vi "Interp2D.vi"(6 "method":i32(ring)=3 items=["nearest", "bilinear", "bicubic", "bicubic spline"], 7 "Fixed Axis":T1, 9 "Interpolation Points":i32=100, 10 "Meas maxima":dbl[](array[numeric]) format="%.1f", 11 "Measured Points":dbl[][](array[numeric]) format="%.2f") -> (1 "Yi":dbl, 2 "Xi":dbl, 3 "max value":dbl)   [LabVIEW 2011]
uses:
  <vilib>/Math Plots/3D Math Plots/3D Surface/3D Surface XCtrl/3D Surface.xctl
  Gen Trav/Route mapping/Axis.ctl
  <vilib>/Analysis/1siggen.llb/Ramp Pattern by Samples.vi
  <vilib>/gmath/interp.llb/Create Mesh Grid (2D) (x,y arrays).vi
  <vilib>/gmath/interp.llb/Interpolate 2D (2d X,Y).vi
  <vilib>/Math Plots/3D Math Plots/3D Surface/3D Surface Datatype/Public/Plot Helper (Matrix).vi
  <vilib>/gmath/NI_Gmath.lvlib
  <vilib>/Analysis/NI_AALBase.lvlib
  <vilib>/Math Plots/3D Math Plots/3D Surface/3D Surface Datatype/3D Surface Datatype.lvclass
panel:
  out "Interpolated Surface":refnum<class "3D Plot Datatype.lvclass">[](xcontrol)
  out "Input Surface":refnum<class "3D Plot Datatype.lvclass">[](xcontrol)
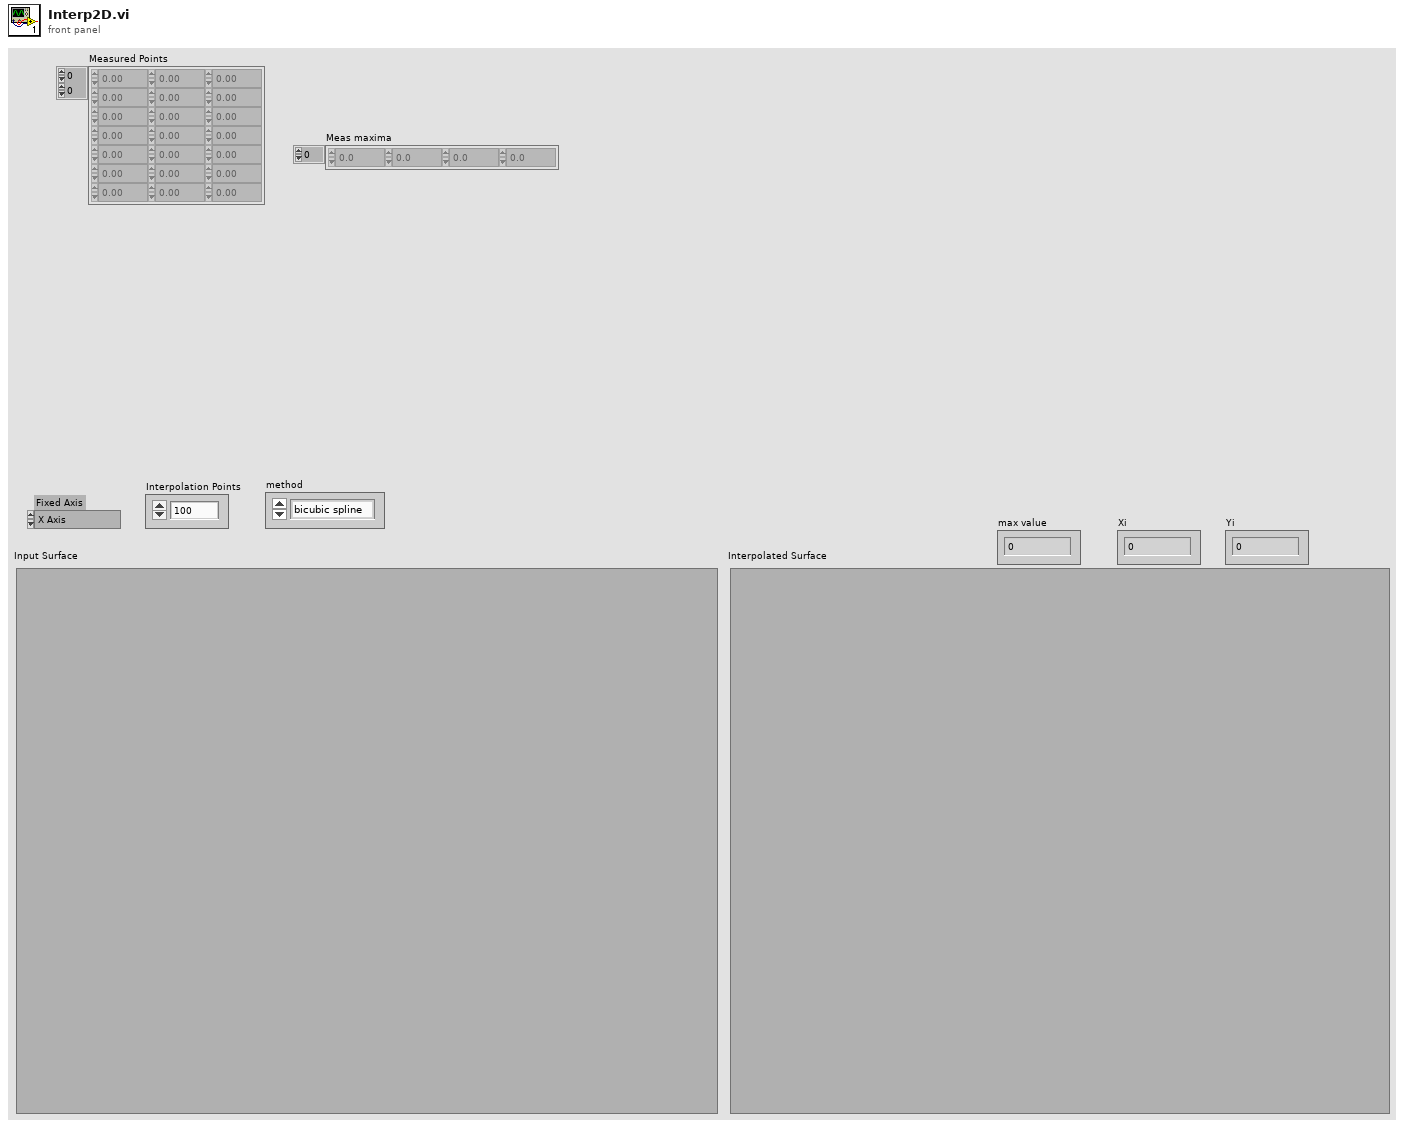
[diagram p1: front panel]
types:
  T1 = typedef "Axis.ctl" = enum16{"X Axis", "X Axis -ve", "Y Axis", "Y Axis -ve", "Z Axis", "Z Axis -ve"}
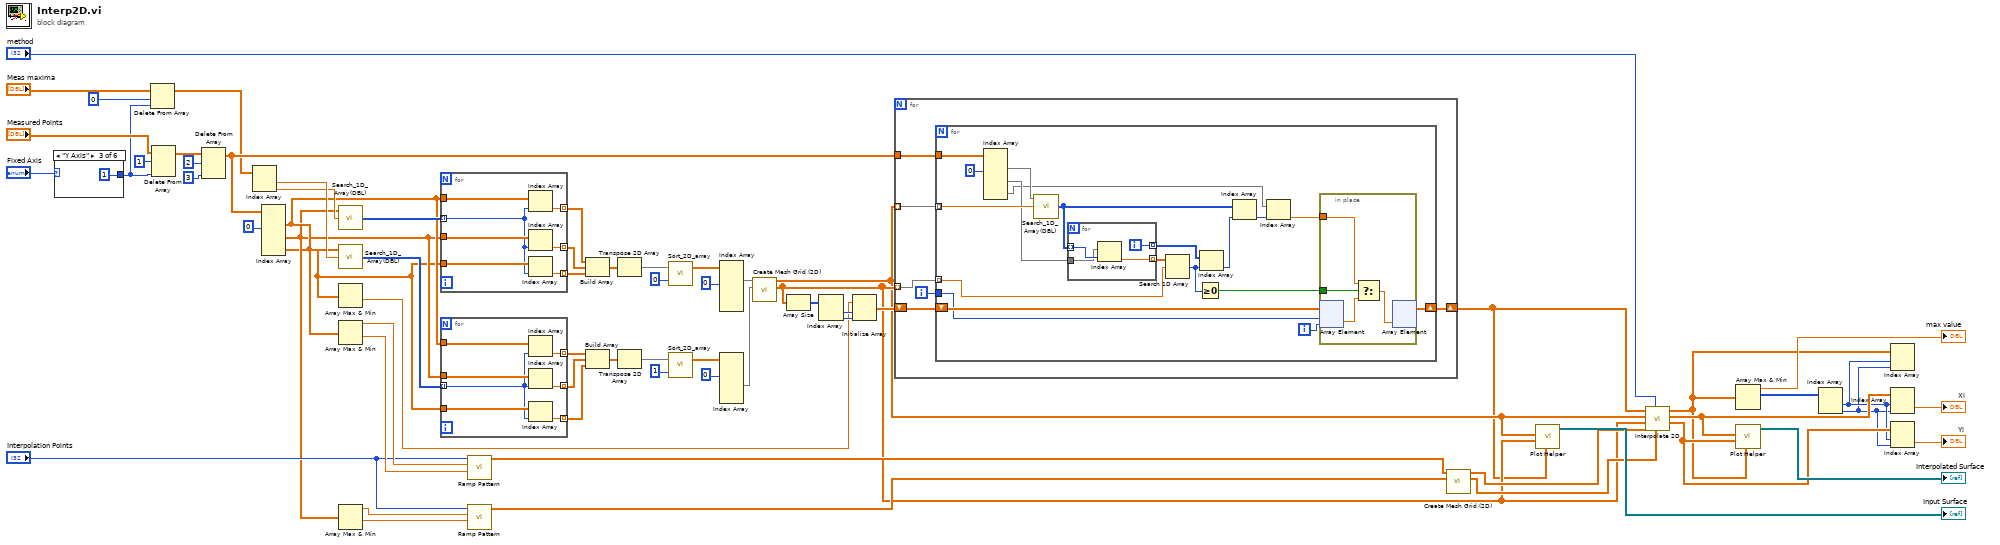
[diagram p0: block diagram]
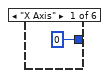
[diagram p2: hidden frame]
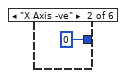
[diagram p3: hidden frame]
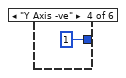
[diagram p4: hidden frame]
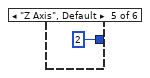
[diagram p5: hidden frame]
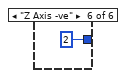
[diagram p6: hidden frame]
diagram:
  n1 = case shown="\"Y Axis\"" "Fixed Axis" {
    tunnel: [0 ("index") 0 ("index") 1 ("index") 1 ("index") 2 ("index") 2 ("index")] -> w1
    frame "X Axis" {
    }
    frame "X Axis -ve" {
    }
    frame "Y Axis" {
    }
    frame "Y Axis -ve" {
    }
    frame "Z Axis", Default {
    }
    frame "Z Axis -ve" {
    }
  }
  n2 = Delete From Array(array="Meas maxima", length=0, index=w1) -> (array with subset deleted=w3:dbl[])  [unwired: 1 out]
  n3 = Delete From Array(array="Measured Points", length=1, index (col)=w1) -> (array with subset deleted=w65:dbl[][])  [unwired: 1 in, 1 out]
  n4 = Delete From Array(array=w65, length=2, index (col)=3 ("disabled index (col)")) -> (array with subset deleted=w16:dbl[][])  [unwired: 1 in, 1 out]
  n5 = Index Array(array=w3) -> (element #1=w55:dbl, element #2=w53:dbl)  [unwired: 2 in]
  n6 = Index Array(array=w16, index (col) #1=0 ("disabled index (col)")) -> (element #1=w41:dbl[], element #2=w40:dbl[], element #3=w15:dbl[])  [unwired: 5 in]
  n7 = call "Search_1D_Array(DBL).vi"("Array"=w40, "Element Data"=w53) -> ("Indicies of Elements"=w52:i32[])  [unwired: 6 in, 1 out]
  n8 = call "Search_1D_Array(DBL).vi"("Array"=w41, "Element Data"=w55) -> ("Indicies of Elements"=w57:i32[])  [unwired: 6 in, 1 out]
  n9 = Array Max & Min(array=w15) -> (min value=w14:dbl)  [unwired: 3 out]
  n10 = Array Max & Min(array=w41) -> (max value=w46:dbl, min value=w45:dbl)  [unwired: 2 out]
  n11 = Array Max & Min(array=w40) -> (max value=w42:dbl, min value=w44:dbl)  [unwired: 2 out]
  n12 = for {
    tunnel: w52 -> [w73] mode=indexing
    tunnel: w41 -> [w79]
    tunnel: w15 -> [w78]
    tunnel: [w77] -> w31 mode=indexing
    tunnel: [w76] -> w50 mode=indexing
    tunnel: [w75] -> w49 mode=indexing
    tunnel: w40 -> [w74]
    n13 = Index Array(array=w79, index=w73) -> (element=w77:dbl)
    n14 = Index Array(array=w74, index=w73) -> (element=w75:dbl)
    n15 = Index Array(array=w78, index=w73) -> (element=w76:dbl)
  }
  n16 = for {
    tunnel: w57 -> [w80] mode=indexing
    tunnel: w41 -> [w86]
    tunnel: w15 -> [w85]
    tunnel: [w84] -> w39 mode=indexing
    tunnel: [w83] -> w54 mode=indexing
    tunnel: [w82] -> w38 mode=indexing
    tunnel: w40 -> [w81]
    n17 = Index Array(array=w86, index=w80) -> (element=w84:dbl)
    n18 = Index Array(array=w81, index=w80) -> (element=w82:dbl)
    n19 = Index Array(array=w85, index=w80) -> (element=w83:dbl)
  }
  n20 = call-poly <vilib>:"Ramp Pattern.vi"("start"=w45, "end"=w46, "samples"="Interpolation Points") -> ("Ramp Pattern"=w25:dbl[])  [unwired: 7 in, 1 out]
  n21 = call-poly <vilib>:"Ramp Pattern.vi"("start"=w44, "end"=w42, "samples"="Interpolation Points") -> ("Ramp Pattern"=w24:dbl[])  [unwired: 7 in, 1 out]
  n22 = Build Array(w31, w49, w50) -> (w51:dbl[][])
  n23 = Build Array(w39, w38, w54) -> (w56:dbl[][])
  n24 = Transpose 2D Array(2D array=w51) -> (transposed array=w47:dbl[][])
  n25 = Transpose 2D Array(2D array=w56) -> (transposed array=w60:dbl[][])
  n26 = call "Sort_2D_array.vi"("Column index to sort on"=0, "unsorted array"=w47) -> ("sorted array"=w32:dbl[][])  [unwired: 1 out]
  n27 = call "Sort_2D_array.vi"("Column index to sort on"=1, "unsorted array"=w60) -> ("sorted array"=w33:dbl[][])  [unwired: 1 out]
  n28 = Index Array(array=w32, index (col) #1=0 ("disabled index (col)")) -> (element #1=w30:dbl[])  [unwired: 5 in, 2 out]
  n29 = Index Array(array=w33, index (col) #1=0 ("disabled index (col)")) -> (element #2=w29:dbl[])  [unwired: 5 in, 2 out]
  n30 = call-poly <vilib>:"Create Mesh Grid (2D).vi"("y domain"=w29, "x domain"=w30) -> ("Y"=w21:dbl[][], "X"=w20:dbl[][])  [unwired: 7 in, 1 out]
  n31 = Array Size(array=w21) -> (size(s)=w37:i32[])
  n32 = Index Array(array=w37) -> (element #1=w36:i32, element #2=w35:i32)  [unwired: 2 in]
  n33 = Initialize Array(w14, w36, w35) -> (w34:dbl[][])
  n34 = for {
    tunnel: w20 -> [w92] mode=indexing
    tunnel: w21 -> [w91] mode=indexing
    tunnel: w16 -> [w90]
    shift-right: [w87] -> w17
    shift-left: w34 -> [w89]
    i -> [w88]
    n35 = for {
      tunnel: w92 -> [w109] mode=indexing
      tunnel: w91 -> [w107] mode=indexing
      tunnel: w90 -> [w111]
      shift-right: [w105] -> w87
      shift-left: w89 -> [w106]
      tunnel: w88 -> [w99]
      i -> [w98]
      n36 = Index Array(array=w111, index (col) #1=0 ("disabled index (col)")) -> (element #1=w108:dbl[], element #2=w104:dbl[], element #3=w102:dbl[])  [unwired: 5 in]
      n37 = call "Search_1D_Array(DBL).vi"("Array"=w108, "Element Data"=w109) -> ("Indicies of Elements"=w94:i32[])  [unwired: 6 in, 1 out]
      n38 = for {
        tunnel: w94 -> [w115] mode=indexing
        tunnel: w104 -> [w114]
        tunnel: [w113] -> w103 mode=indexing
        tunnel: [w112] -> w97 mode=indexing
        i -> [w112]
        n39 = Index Array(array=w114, index=w115) -> (element=w113:dbl)
      }
      n40 = Search 1D Array(1D array=w103, element=w107) -> (index of element=w96:i32)  [unwired: 1 in]
      n41 = Greater Or Equal To 0?(x=w96) -> (x >= 0?=w100:bool)
      n42 = Index Array(array=w97, index=w96) -> (element=w95:i32)
      n43 = Index Array(array=w94, index=w95) -> (element=w93:i32)
      n44 = Index Array(array=w102, index=w93) -> (element=w101:dbl)
      n45 = in-place {
        in-place-border: w101 -> [w118]
        in-place-border: w100 -> [w119]
        n46 = in-place-array #1(w106, w99, w98) -> (w117:dbl)
        n47 = Select(t=w118, s=w119, f=w117) -> (s? t:f=w116:dbl)
        n48 = in-place-array #1(w116) -> (w105:dbl[][])  [unwired: 2 out]
      }
    }
  }
  n49 = call-poly <vilib>:"Create Mesh Grid (2D).vi"("y domain"=w24, "x domain"=w25) -> ("Y"=w22:dbl[][], "X"=w23:dbl[][])  [unwired: 7 in, 1 out]
  n50 = call-poly <vilib>:"Plot Helper.vi"("z matrix"=w17, "y matrix"=w21, "x matrix"=w20) -> ("3D Plot lvclass Array out"=→"Input Surface":refnum<class "3D Plot Datatype.lvclass">[])  [unwired: 3 in, 5 out]
  n51 = call-poly <vilib>:"Interpolate 2D.vi"("yi"=w22, "method"="method", "xi"=w23, "Y"=w21, "X"=w20, "Z"=w17) -> ("yi used"=w11:dbl[][], "xi used"=w12:dbl[][], "zi"=w5:dbl[][])  [unwired: 2 in, 1 out]
  n52 = Array Max & Min(array=w5) -> (max value=→"max value":dbl, max index (indices)=w13:i32[])  [unwired: 2 out]
  n53 = call-poly <vilib>:"Plot Helper.vi"("z matrix"=w5, "y matrix"=w11, "x matrix"=w12) -> ("3D Plot lvclass Array out"=→"Interpolated Surface":refnum<class "3D Plot Datatype.lvclass">[])  [unwired: 3 in, 5 out]
  n54 = Index Array(array=w13) -> (element #1=w7:i32, element #2=w6:i32)  [unwired: 2 in]
  n55 = Index Array(array=w5, index (row)=w7, index (col)=w6) -> ()  [unwired: 1 out]
  n56 = Index Array(array=w12, index (row)=w7, index (col)=w6) -> (element=→"Xi":dbl)
  n57 = Index Array(array=w11, index (row)=w7, index (col)=w6) -> (element=→"Yi":dbl)
